vi "test Loopback_Acyclic Messages.vi"(8 "error in":errorcluster, 11 "TestCase in":refnum<class "SingleCore.lvclass">) -> (0 "error out":errorcluster, 3 "TestCase out":refnum<class "SingleCore.lvclass">)   [LabVIEW 2020, in "SingleCore.lvclass"]
uses:
  SingleCore.lvclass
  C:/Git/niveristand-custom-device-testing-tools/VeriStandTestCase/VeriStandTestCase.lvclass
  4b06c685-66bb-4135-9ad1-d89a50a95502.vi
  <vilib>/numeric/Random Number (Range) I64.vi
  <vilib>/numeric/sub_Random U32.vi
  <vilib>/NI VeriStand/Execution/Workspace/NI VeriStand - Set Multiple Channel Values.vi
  <vilib>/addons/_JKI Toolkits/VI Tester/TestCase.llb/TestCase.lvclass
  <vilib>/NI VeriStand/Execution/Workspace/NI_VS Workspace ExecutionAPI.lvlib
  C:/Program Files (x86)/National Instruments/LabVIEW 2020/vi.lib/addons/_JKI Toolkits/VI Tester/TestCase.llb/TestCase.lvclass
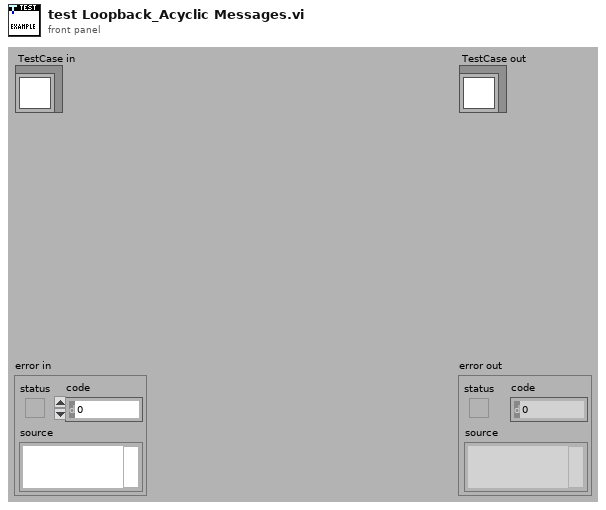
[diagram p1: front panel]
types:
  T1 = typedef "NI_VS Workspace ExecutionAPI.lvlib/WorkspaceAPI.ctl" = refnum<k24>
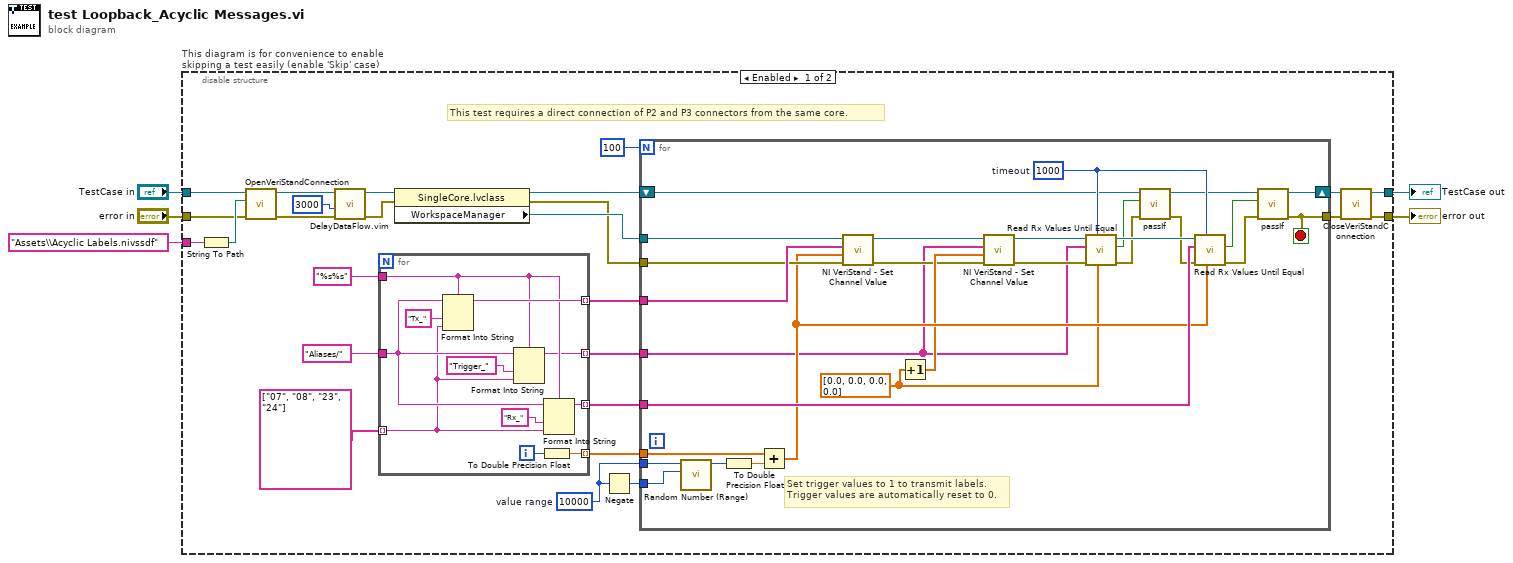
[diagram p0: block diagram]
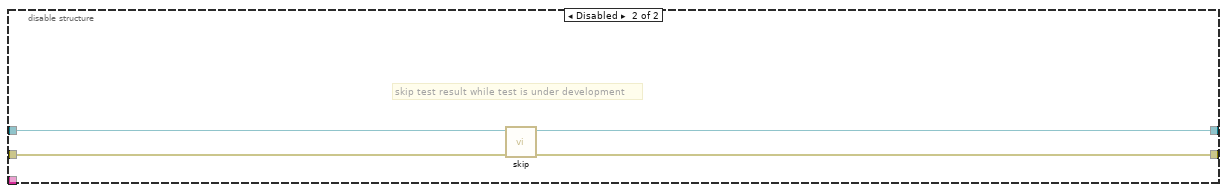
[diagram p2: hidden frame]
diagram:
  n1 = disable-structure "This diagram is for convenience to enable skipping a test easily (enable 'Skip' case)" shown="Enabled" {
    disable-tunnel: "TestCase in" -> [w25 w73]
    disable-tunnel: [w22 w71] -> w2
    disable-tunnel: [w21 w72] -> w4
    disable-tunnel: "error in" -> [w24 w70]
    disable-tunnel: "Assets\\Acyclic Labels.nivssdf" ("Channel") -> [w23 _]
    frame Enabled {
      w19 = i64 10000  # value range
      # "This test requires a direct connection of P2 and P3 connectors from the same core."
      n2 = String To Path(string=w23) -> (path=w26:path)
      n3 = call-dynamic "OpenVeriStandConnection.vi"("error in (no error)"=w24, "System Definition File"=w26, "VeriStand Test Case in"=w25) -> ("error out"=w28:errorcluster, "VeriStand Test Case out"=w30:refnum<class "SingleCore.lvclass">)  [unwired: 6 in, 1 out]
      n4 = call "DelayDataFlow.vim"("value in"=w28, "milliseconds to wait"=u32 3000) -> ("value out"=w27:errorcluster)  [unwired: 2 in, 1 out]
      n5 = for {
        tunnel: [w69] -> w17 mode=indexing
        tunnel: [w64] -> w14 mode=indexing
        tunnel: [w68] -> w20 mode=indexing
        tunnel: "Aliases/" ("Channel") -> [w63]
        tunnel: string[] ["07", "08", "23", "24"] -> [w62] mode=indexing
        tunnel: "%s%s" ("format string") -> [w60]
        tunnel: [w59] -> w6 mode=indexing
        i -> [w67]
        n6 = Format Into String(format string=w60, initial string=w63, "Tx_" ("input 1"), w62) -> (resulting string=w69:string)  [unwired: 1 in, 1 out]
        n7 = Format Into String(format string=w60, initial string=w63, "Trigger_" ("input 1"), w62) -> (resulting string=w59:string)  [unwired: 1 in, 1 out]
        n8 = To Double Precision Float(number=w67) -> (double precision float=w68:dbl)
        n9 = Format Into String(format string=w60, initial string=w63, "Rx_" ("input 1"), w62) -> (resulting string=w64:string)  [unwired: 1 in, 1 out]
      }
      n10 = property class="SingleCore.lvclass"(reference=w30, error in=w27) -> (reference out=w13:refnum<class "SingleCore.lvclass">, error out=w15:errorcluster, "WorkspaceManager"=w16:T1)
      n11 = Negate(x=w19) -> (-x=w18:i64)
      n12 = for {
        N: 100 -> [_]
        tunnel: w20 -> [w56]
        tunnel: w19 -> [w55]
        tunnel: w18 -> [w54]
        tunnel: w17 -> [w53]
        tunnel: w16 -> [w52]
        tunnel: w15 -> [w51]
        tunnel: w14 -> [w50]
        shift-right: [w48] -> w12
        shift-left: w13 -> [w32]
        tunnel: [w46] -> w11
        tunnel: w6 -> [w38]
        stop <- w46 stop-if-true
        w37 = dbl[] [0.0, 0.0, 0.0, 0.0]
        w36 = 1000  # timeout
        # "Set trigger values to 1 to transmit labels. \nTrigger values are automatically reset to 0."
        n13 = call-poly <vilib>:"Random Number (Range).vi"("lower bound (-100)"=w54, "upper bound (100)"=w55) -> ("number"=w58:i64)  [unwired: 9 in]
        n14 = To Double Precision Float(number=w58) -> (double precision float=w57:dbl)
        n15 = Add(x=w56, y=w57) -> (x+y=w47:dbl[])
        n16 = call-poly <vilib>:"NI VeriStand - Set Channel Value.vi"("error in (no error)"=w51, "Values"=w47, "Channels"=w53, "WorkspaceManager in"=w52) -> ("error out"=w42:errorcluster, "WorkspaceManager out"=w43:T1)  [unwired: 6 in]
        n17 = Increment(x=w37) -> (x+1=w44:dbl[])
        n18 = call-poly <vilib>:"NI VeriStand - Set Channel Value.vi"("error in (no error)"=w42, "Values"=w44, "Channels"=w38, "WorkspaceManager in"=w43) -> ("error out"=w40:errorcluster, "WorkspaceManager out"=w41:T1)  [unwired: 6 in]
        n19 = call "Read Rx Values Until Equal.vi"("expected values"=w37, "timeout (1000 ms)"=w36, "error in"=w40, "Rx aliases"=w38, "workspace manager in"=w41) -> ("error out"=w33:errorcluster, "values equal expected"=w31:bool, "workspace manager out"=w39:T1)  [unwired: 4 in]
        n20 = call-dynamic "passIf.vi"("error in (no error)"=w33, "pass"=w31, "TestCase in"=w32) -> ("error out"=w34:errorcluster, "TestCase out"=w35:refnum<class "SingleCore.lvclass">)  [unwired: 7 in]
        n21 = call "Read Rx Values Until Equal.vi"("expected values"=w47, "timeout (1000 ms)"=w36, "error in"=w34, "Rx aliases"=w50, "workspace manager in"=w39) -> ("error out"=w49:errorcluster, "values equal expected"=w45:bool)  [unwired: 4 in, 1 out]
        n22 = call-dynamic "passIf.vi"("error in (no error)"=w49, "pass"=w45, "TestCase in"=w35) -> ("error out"=w46:errorcluster, "TestCase out"=w48:refnum<class "SingleCore.lvclass">)  [unwired: 7 in]
      }
      n23 = call-dynamic "CloseVeriStandConnection.vi"("error in (no error)"=w11, "VeriStand Test Case in"=w12) -> ("error out"=w21:errorcluster, "VeriStand Test Case out"=w22:refnum<class "SingleCore.lvclass">)  [unwired: 8 in]
    }
    frame Disabled {
      # "skip test result while test is under development"
      n24 = call <vilib>:"skip.vi"("error in (no error)"=w70, "TestCase in"=w73) -> ("error out"=w72:errorcluster, "TestCase out"=w71:refnum<class "SingleCore.lvclass">)  [unwired: 8 in]
    }
  }
  "error out" <- w4
  "TestCase out" <- w2
